vi "SERIAL_YPRCGlobal.vi"(11 "YPRH":T1) -> (0 "Last Update":dbl, 3 "YPRH":T1)   [LabVIEW 2016, in "navX-MXP IMU.lvlib"]
uses:
  navX-MXP IMU.lvlib
  COMMON/TypeDefs/navX YPRH Data.ctl
  <vilib>/Rock Robotics/SystemInterfaces/Utilities/FPGA_UtilitiesRead LocalTime.vi
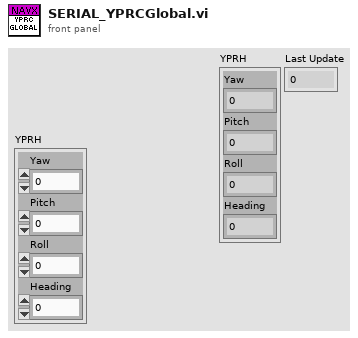
[diagram p1: front panel]
types:
  T1 = typedef "navX-MXP IMU.lvlib/navX YPRH Data.ctl" = cluster{"Yaw":dbl, "Pitch":dbl, "Roll":dbl, "Heading":dbl}
  T2 = cluster{"Yaw":bool, "Pitch":bool, "Roll":bool, "Heading":bool}
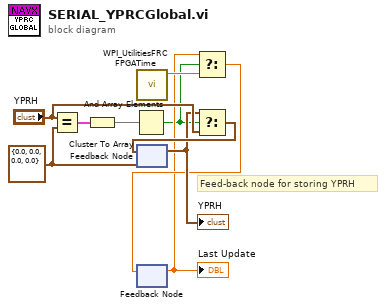
[diagram p0: block diagram]
diagram:
  w10 = T1 {"Yaw"=0.0, "Pitch"=0.0, "Roll"=0.0, "Heading"=0.0} ("YPR Update")
  # "Feed-back node for storing YPRH"
  n1 = Equal?(x="YPRH", y=w10) -> (x = y?=w9:T2)
  n2 = Cluster To Array(cluster=w9) -> (array=w8:bool[])
  n3 = And Array Elements(Boolean array=w8) -> (logical AND=w1:bool)
  n4 = call <vilib>:"WPI_UtilitiesFRC FPGATime.vi"() -> ("FPGA Time"=w4:dbl)  [unwired: 10 in, 1 out]
  n5 = feedback #1(w10) -> (w5:T1)
  "YPRH" <- w5
  n6 = feedback #2() -> (w2:dbl)  [unwired: 1 in]
  "Last Update" <- w2
  n7 = Select(t=w2, s=w1, f=w4) -> (s? t:f=w3:dbl)
  n8 = feedback-in #2(w3) -> ()
  n9 = Select(t=w5, s=w1, f="YPRH") -> (s? t:f=w6:T1)
  n10 = feedback-in #1(w6) -> ()
